vi "kalmanError.vi"(10 "Kalman Error ID":i32, 11 "IA state":T1={"our_robots"=[], "enemy_robots"=[], "balls"=[], "geometry"={"line_width"=0, "field_length"=0, "field_width"=0, "boundary_width"=0, "referee_width"=0, "goal_width"=0, "goal_depth"=0, "goal_wall_width"=0, "center_circle_radius"=0, "defense_radius"=0, "defense_stretch"=0, "free_kick_from_defense_dist"=0, "penalty_spot_from_field_line_dist"=0, "penalty_line_from_spot_dist"=0}, "IA Judge"={"stage"="", "command"="", "our_goalie_id"=0.0, "enemy_goalie_id"=0.0, "command enum"=enum."Halt", "Time"=enum."Azul"}, "Received Timestamp"=timestamp(0 s since 1904-01-01), "Events"={"Touch"=FALSE, "Ball out"=FALSE, "id touch"=0.0, "Ball out of \nVision"=FALSE, "Ball inside \nGoalie area"=FALSE, "Robot not responding"=FALSE, "Robots responding status"=[1.0, 1.0, 1.0, 1.0, 1.0, 1.0], "Enemy Ball \nPossession"=FALSE, "Pass State"=FALSE, "id end of pass"=0.0, "Kick"=FALSE, "Id ini Possession"=0.0, "Ball Possesion"=FALSE, "Id Possesion"=0.0}}) -> (3 "Kalman Error Histogram":cluster{dbl[], dbl[]}(graph))   [LabVIEW 2017]
uses:
  Core/AI Input.ctl
  Core/AI Robot.ctl
  Intel/Functions Enum.ctl
  Intel/AttackerStates.ctl
  Core/AI Ball.ctl
  Core/Field Size.ctl
  Core/AI Judge.ctl
  Intel/Command Enum.ctl
  Util/Events/Events.ctl
  <vilib>/Analysis/coordinate.llb/2D Cartesian Coordinate Rotation (Scalar).vi
  <vilib>/Analysis/NI_AALPro.lvlib
panel:
  in  "Erro máximo":i32=5
  in  "Intervalos de erro":i32=10
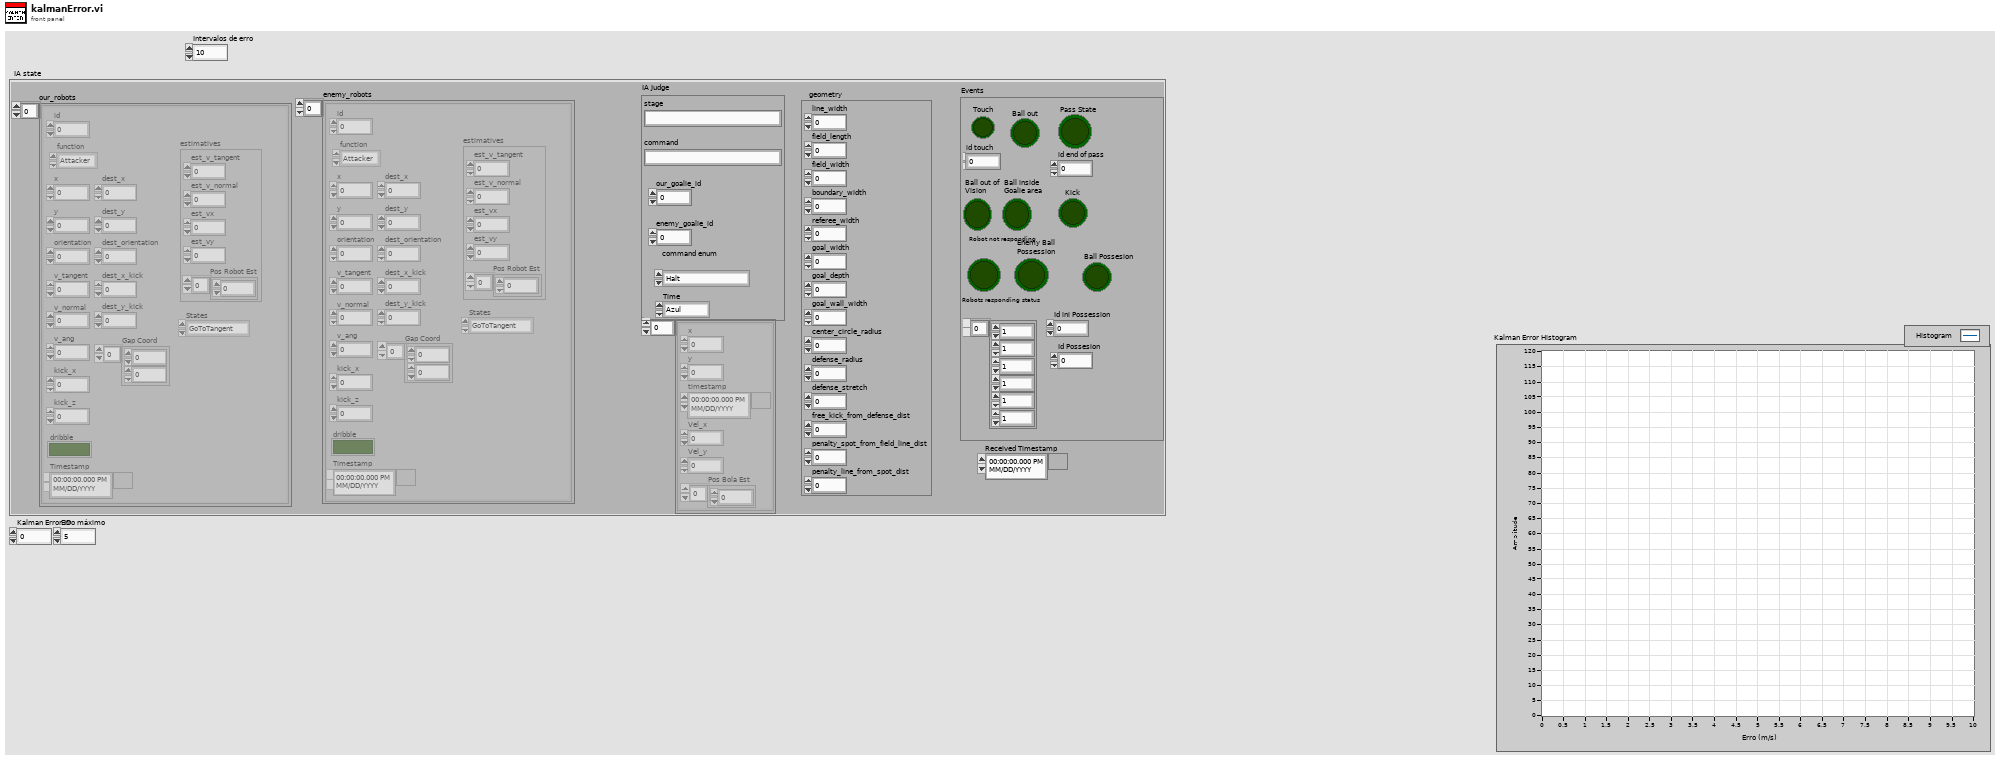
[diagram p1: front panel]
types:
  T1 = typedef "AI Input.ctl" = cluster{"our_robots":T2[], "enemy_robots":T2[], "balls":T5[], "geometry":T6, "IA Judge":T7, "Received Timestamp":timestamp, "Events":T9}
  T2 = typedef "AI Robot.ctl" = cluster{"id":u32, "function":T3, "x":dbl, "y":dbl, "orientation":dbl, "v_tangent":dbl, "v_normal":dbl, "v_ang":dbl, "kick_x":dbl, "kick_z":dbl, "dribble":bool, "Timestamp":timestamp, "dest_x":dbl, "dest_y":dbl, "dest_orientation":dbl, "estimatives":cluster{"est_v_tangent":dbl, "est_v_normal":dbl, "est_vx":dbl, "est_vy":dbl, "Pos Robot Est":dbl[]}, "dest_x_kick":dbl, "dest_y_kick":dbl, "Gap Coord":dbl[], "States":T4}
  T3 = typedef "Functions Enum.ctl" = enum16{"Attacker", "Goalie", "Defender", "Striker", "Goto 0", "Dummy", "Kicker", "ZigZag"}
  T4 = typedef "AttackerStates.ctl" = enum16{"Pass", "GoToTangent", "BallGetting", "GoToKick", ""}
  T5 = typedef "AI Ball.ctl" = cluster{"x":dbl, "y":dbl, "timestamp":timestamp, "Vel_x":dbl, "Vel_y":dbl, "Pos Bola Est":dbl[]}
  T6 = typedef "Field Size.ctl" = cluster{"line_width":u32, "field_length":u32, "field_width":u32, "boundary_width":u32, "referee_width":u32, "goal_width":u32, "goal_depth":u32, "goal_wall_width":u32, "center_circle_radius":u32, "defense_radius":u32, "defense_stretch":u32, "free_kick_from_defense_dist":u32, "penalty_spot_from_field_line_dist":u32, "penalty_line_from_spot_dist":u32}
  T7 = typedef "AI Judge.ctl" = cluster{"stage":string, "command":string, "our_goalie_id":dbl, "enemy_goalie_id":dbl, "command enum":T8, "Time":enum16{"Azul", "Amarelo"}}
  T8 = typedef "Command Enum.ctl" = enum16{"Halt", "Stop", "Force Start", "PKA Normal Start", "Prepare Kickoff Ally", "PKE Normal Start", "Prepare Kickoff Enemy", "Prepare Penalty Ally", "PPA Normal Start", "Prepare Penalty Enemy", "PPE Normal Start", "Direct Free Enemy", "Direct Free Ally", "Indirect Free Enemy", "Indirect Free Ally", "Timeout Enemy", "Timeout Ally", "Goal Enemy", "Goal Ally", "Ball Placement Enemy", "Ball Placement Ally", "Normal Half Time", "Extra Time Break", "Extra Half Time", "None", "Post Game"}
  T9 = typedef "Events.ctl" = cluster{"Touch":bool, "Ball out":bool, "id touch":dbl, "Ball out of \nVision":bool, "Ball inside \nGoalie area":bool, "Robot not responding":bool, "Robots responding status":dbl[], "Enemy Ball \nPossession":bool, "Pass State":bool, "id end of pass":dbl, "Kick":bool, "Id ini Possession":dbl, "Ball Possesion":bool, "Id Possesion":dbl}
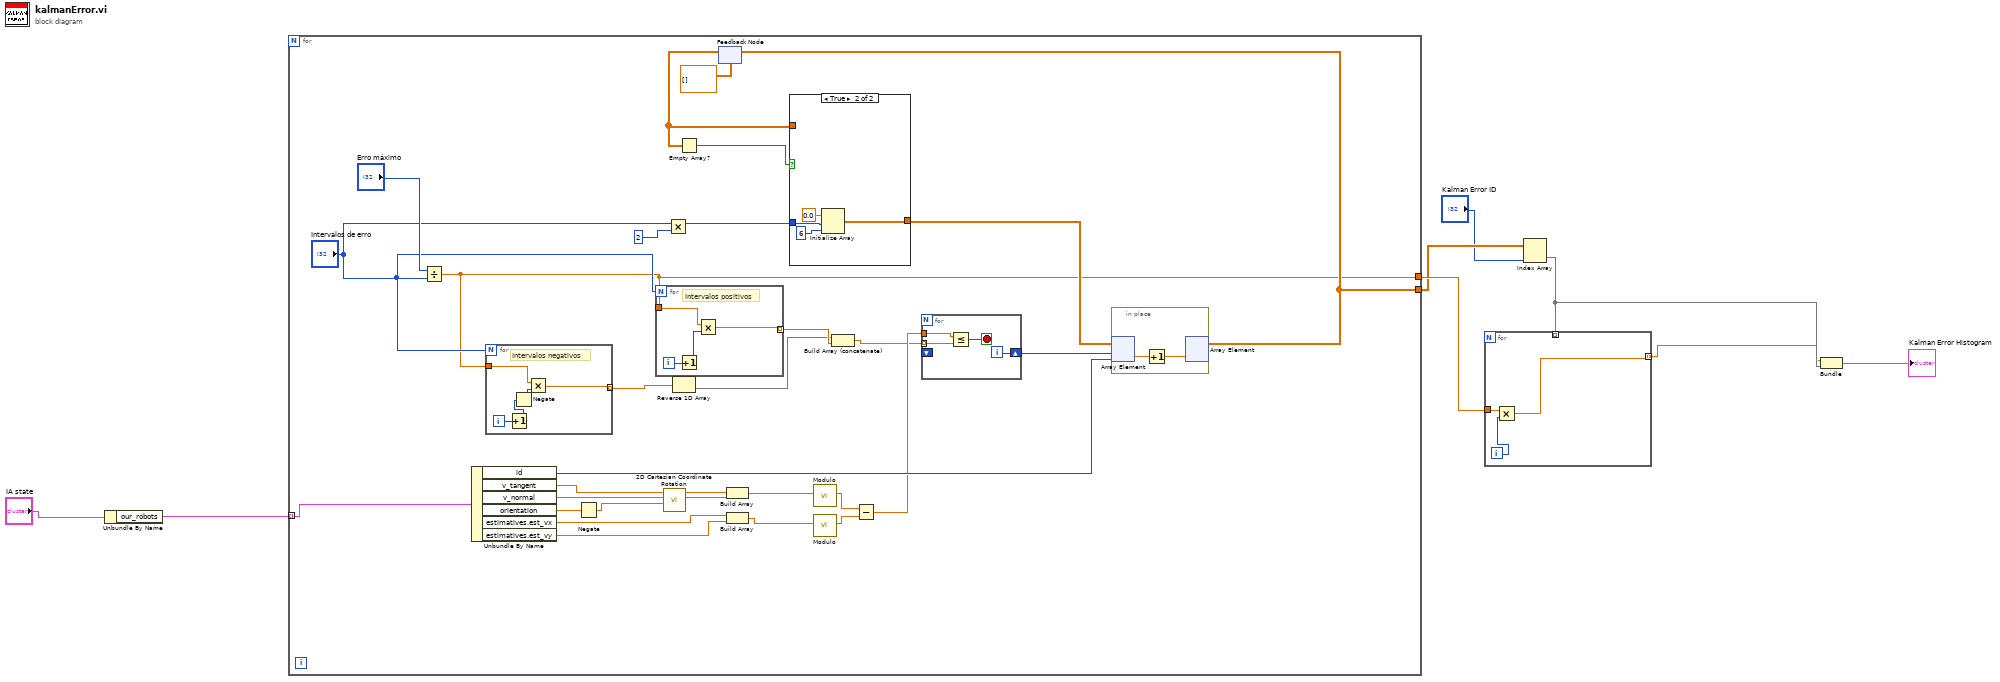
[diagram p0: block diagram]
diagram:
  n1 = Unbundle By Name("IA state") -> ("our_robots"=w7:T2[])
  n2 = for {
    tunnel: w7 -> [w38] mode=indexing
    tunnel: [w10] -> w5
    tunnel: [w9] -> w6
    n3 = Divide(x="Erro máximo", y="Intervalos de erro") -> (x/y=w9:dbl)
    n4 = Unbundle By Name(w38) -> ("id"=w20:u32, "v_tangent"=w37:dbl, "v_normal"=w36:dbl, "orientation"=w35:dbl, "estimatives.est_vx"=w31:dbl, "estimatives.est_vy"=w30:dbl)
    n5 = for {
      N: "Intervalos de erro" -> [_]
      tunnel: w9 -> [w43]
      tunnel: [w42] -> w15 mode=indexing
      i -> [w41]
      # "Intervalos negativos"
      n6 = Increment(x=w41) -> (x+1=w40:i32)
      n7 = Negate(x=w40) -> (-x=w39:i32)
      n8 = Multiply(x=w43, y=w39) -> (x*y=w42:dbl)
    }
    n9 = Negate(x=w35) -> (-x=w34:dbl)
    n10 = for {
      N: "Intervalos de erro" -> [_]
      tunnel: w9 -> [w54]
      tunnel: [w53] -> w14 mode=indexing
      i -> [w52]
      # "Intervalos positivos"
      n11 = Increment(x=w52) -> (x+1=w51:i32)
      n12 = Multiply(x=w54, y=w51) -> (x*y=w53:dbl)
    }
    n13 = call-poly <vilib>:"2D Cartesian Coordinate Rotation.vi"("theta"=w34, "y"=w36, "x"=w37) -> ("y out"=w32:dbl, "x out"=w33:dbl)  [unwired: 6 in, 1 out]
    n14 = Multiply(x="Intervalos de erro", y=2) -> (x*y=w12:i32)
    n15 = Reverse 1D Array(array=w15) -> (reversed array=w13:dbl[])
    n16 = feedback #1(dbl[][] []) -> (w24:dbl[][])
    n17 = Empty Array?(array=w24) -> (empty?=w21:bool)
    n18 = Build Array(w33, w32) -> (w29:dbl[])
    n19 = Build Array(w31, w30) -> (w28:dbl[])
    n20 = case shown="True" w21 {
      tunnel: w24 -> [w46 _]
      tunnel: [w46 w48] -> w22
      tunnel: w12 -> [_ w47]
      frame False {
      }
      frame True {
        n21 = Initialize Array(0.0 ("element"), w47, 6 ("dimension size")) -> (w48:dbl[][])
      }
    }
    n22 = call "Modulo.vi"("2D vector"=w29) -> ("Modulo"=w26:dbl)  [unwired: 10 in]
    n23 = call "Modulo.vi"("2D vector"=w28) -> ("Modulo"=w27:dbl)  [unwired: 10 in]
    n24 = Build Array (concatenate)(w13, w14) -> (w17:dbl[])
    n25 = Subtract(x=w26, y=w27) -> (x-y=w18:dbl)
    n26 = for {
      shift-right: [w57] -> w19
      shift-left: _ -> [_]
      tunnel: w18 -> [w56]
      tunnel: w17 -> [w55] mode=indexing
      i -> [w57]
      stop <- w58 stop-if-true
      n27 = Less Or Equal?(x=w56, y=w55) -> (x <= y?=w58:bool)
    }
    n28 = in-place {
      n29 = in-place-array #2(w22, w19, w20) -> (w45:dbl)
      n30 = Increment(x=w45) -> (x+1=w44:dbl)
      n31 = in-place-array #2(w44) -> (w10:dbl[][])  [unwired: 2 out]
    }
    n32 = feedback-in #1(w10) -> ()
  }
  n33 = Index Array(array=w5, index (col)="Kalman Error ID") -> (element=w3:dbl[])  [unwired: 1 in]
  n34 = for {
    tunnel: [w60] -> w1 mode=indexing
    tunnel: w6 -> [w59]
    tunnel: w3 -> [_] mode=indexing
    i -> [w61]
    n35 = Multiply(x=w59, y=w61) -> (x*y=w60:dbl)
  }
  n36 = Bundle(w1, w3) -> (→"Kalman Error Histogram":cluster{dbl[], dbl[]})  [unwired: 1 in]
